vi "Page_Source_Get_Inclusion_Types.vi"(8 "error in (no error)":errorcluster, 11 "AB_PackedLibrary in":refnum<class "AB_PackedLibrary.lvclass">) -> (0 "error out":errorcluster, 2 "supportedFunctions":T1, 3 "AB_PackedLibrary out":refnum<class "AB_PackedLibrary.lvclass">)   [LabVIEW 2020, in "AB_PackedLibrary.lvclass"]
uses:
  <vilib>/AppBuilder/AB_Classes/PackedLib/AB_PackedLibrary.lvclass
  <resource>/Framework/Providers/Builds/AppBuilder/AB_UI_Page_Source_Files_supportedFunctions.ctl
  <vilib>/AppBuilder/AB_Source_Inclusion.ctl
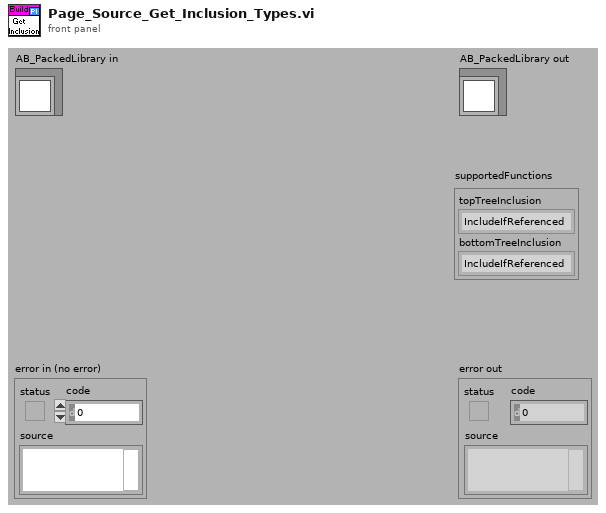
[diagram p1: front panel]
types:
  T1 = typedef "AB_UI_Page_Source_Files_supportedFunctions.ctl" = cluster{"topTreeInclusion":T2, "bottomTreeInclusion":T2}
  T2 = typedef "AB_Source_Inclusion.ctl" = enum16{"IncludeIfReferenced", "Include", "Exclude", "TopLevel"}
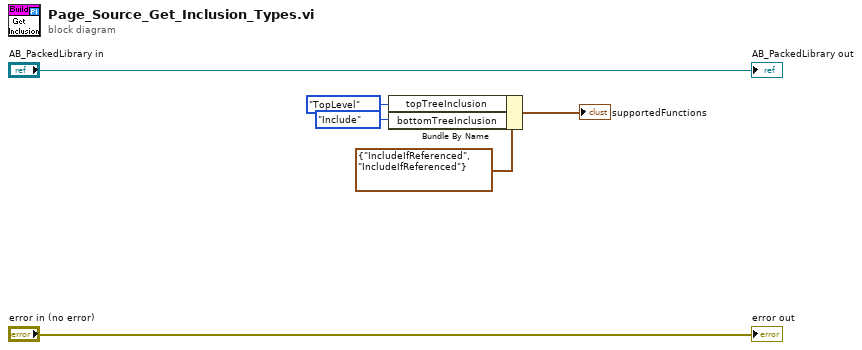
[diagram p0: block diagram]
diagram:
  n1 = Bundle By Name(cluster=T1 {"topTreeInclusion"=enum."IncludeIfReferenced", "bottomTreeInclusion"=enum."IncludeIfReferenced"} ("supportedFunctions"), "topTreeInclusion"=AB_Source_Inclusion."TopLevel", "bottomTreeInclusion"=AB_Source_Inclusion."Include") -> (→"supportedFunctions":T1)
  "error out" <- "error in (no error)"
  "AB_PackedLibrary out" <- "AB_PackedLibrary in"
